vi "solar_tcp Bits Set.vi"(8 "Value (Binary) [Byte Aligned]":string, 9 "Bit Size (0..64)":i32=32, 10 "Bit Offset (0)":i32, 11 "Buffered Data in":string) -> (3 "Data out":string)   [LabVIEW 2018]
doc: "This sets the byte aligned <b>Value</b> into the <b>Buffered Data</b> specified by <b>Bit Length</b> and <b>Bit Size</b>. The <b>Buffered Data</b> must be padded."
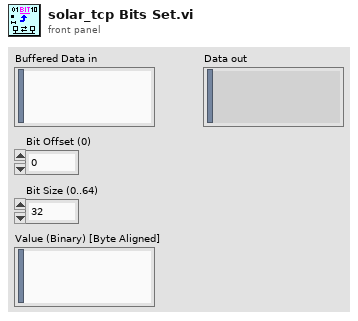
[diagram p1: front panel]
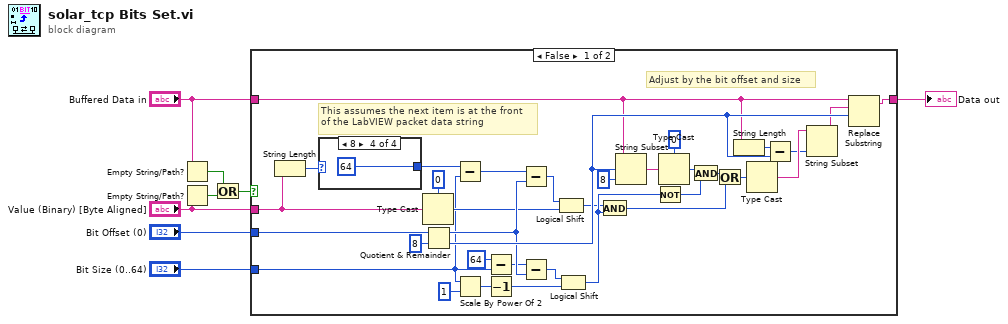
[diagram p0: block diagram]
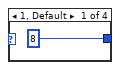
[diagram p2: hidden frame]
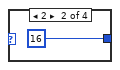
[diagram p3: hidden frame]
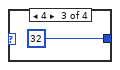
[diagram p4: hidden frame]
diagram:
  n1 = Empty String/Path?(string/path="Buffered Data in") -> (empty?=w1:bool)
  n2 = Empty String/Path?(string/path="Value (Binary) [Byte Aligned]") -> (empty?=w4:bool)
  n3 = Or(x=w1, y=w4) -> (x .or. y?=w3:bool)
  n4 = case shown="False" w3 {
    tunnel: "Buffered Data in" -> [w14 w47]
    tunnel: [w13 w47] -> w8
    tunnel: "Bit Offset (0)" -> [w12 _]
    tunnel: "Value (Binary) [Byte Aligned]" -> [w11 _]
    tunnel: "Bit Size (0..64)" -> [w9 _]
    frame False {
      # "Adjust by the bit offset and size"
      # "This assumes the next item is at the front\nof the LabVIEW packet data string"
      n5 = String Length(string=w11) -> (length=w38:i32)
      n6 = case shown="8" w38 {
        tunnel: [8 16 32 64] -> w20
        frame 1, Default {
        }
        frame 2 {
        }
        frame 4 {
        }
        frame 8 {
        }
      }
      n7 = Type Cast(type=u64 0, x=w11) -> (*(type *) &x=w39:u64)
      n8 = Quotient & Remainder(x=w12, y=8) -> (x-y*floor(x/y)=w40:i32, floor(x/y)=w41:i32)
      n9 = Subtract(x=w20, y=w9) -> (x-y=w19:i32)
      n10 = Scale By Power Of 2(n=w9, x=u64 1) -> (x*2^n=w27:u64)
      n11 = Subtract(x=64, y=w9) -> (x-y=w16:i32)
      n12 = Decrement(x=w27) -> (x-1=w28:u64)
      n13 = Subtract(x=w19, y=w40) -> (x-y=w18:i32)
      n14 = Subtract(x=w16, y=w40) -> (x-y=w15:i32)
      n15 = Logical Shift(y=w18, x=w39) -> (x << y=w33:u64)
      n16 = Logical Shift(y=w15, x=w28) -> (x << y=w34:u64)
      n17 = And(x=w33, y=w34) -> (x .and. y?=w10:u64)
      n18 = String Subset(string=w14, offset (0)=w41, length (rest)=8 ("length (rest)")) -> (substring=w25:string)
      n19 = Not(x=w34) -> (.not. x?=w30:u64)
      n20 = Type Cast(type=u64 0, x=w25) -> (*(type *) &x=w29:u64)
      n21 = And(x=w29, y=w30) -> (x .and. y?=w31:u64)
      n22 = Or(x=w31, y=w10) -> (x .or. y?=w32:u64)
      n23 = String Length(string=w14) -> (length=w22:i32)
      n24 = Type Cast(x=w32) -> (*(type *) &x=w35:string)  [unwired: 1 in]
      n25 = Subtract(x=w22, y=w41) -> (x-y=w21:i32)
      n26 = String Subset(string=w35, length (rest)=w21) -> (substring=w36:string)  [unwired: 1 in]
      n27 = Replace Substring(3:w41, 4:w36, 5:w14) -> (1:w13:string)  [unwired: 2 out]
    }
    frame True {
    }
  }
  "Data out" <- w8
